vi "Read Queue of Self Attributes.vi"(11 "Base Setup in":refnum<class "Base Setup.lvclass">) -> (2 "Queue of Self Attributes":refnum<queue>)   [LabVIEW 2025, in "jettl.lvlib" / "Setup.lvlib" / "Base Setup.lvclass"]
uses:
  Base Setup.lvclass
  Base Setup.lvclass/Base Setup.ctl
  Attributes/Attributes/Attributes.lvclass
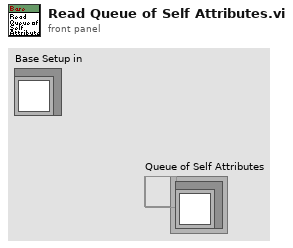
[diagram p1: front panel]
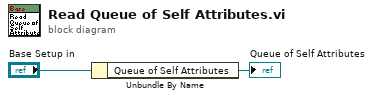
[diagram p0: block diagram]
diagram:
  n1 = Unbundle By Name("Base Setup in") -> ("Queue of Self Attributes"=→"Queue of Self Attributes":refnum<queue>)
